vi "drum-seq-pulse-test.vi"() -> ()   [LabVIEW 2019]
uses:
  <vilib>/Rock Robotics/WPI/ThirdParty/JAS_Junk/TrajLib/Enum/DrumSequence_Step_Enum.ctl
  <vilib>/Rock Robotics/WPI/ThirdParty/JAS_Junk/TrajLib/Enum/DrumSequence_State_Enum.ctl
  <vilib>/Rock Robotics/WPI/ThirdParty/JAS_Junk/TrajLib/VI/BoolCmd_Recv_Internal.vi
  <vilib>/Rock Robotics/WPI/ThirdParty/JAS_Junk/TrajLib/VI/DigSeqLogic_Edge_On.vi
  <vilib>/Rock Robotics/WPI/ThirdParty/JAS_Junk/TrajLib/VI/BoolCmd_Send_Internal.vi
  <vilib>/Rock Robotics/WPI/ThirdParty/JAS_Junk/TrajLib/VI/BoolCmd_ObtainQueue.vi
  <vilib>/Rock Robotics/WPI/ThirdParty/JAS_Junk/TrajLib/Trajectory_Library.lvlib
panel:
  out "DrumSeq_State_ENUM":T1
  out "Loop Count":i32
  out "Output 2":bool
  out "Output 1":bool
  out "Error":bool
  out "Ready":bool
  out "Seq  Active":bool
  out "Step Number":T2=enum."Initialize"
  out "can recv":bool
  out "error out 7":errorcluster
  out "error out 6":errorcluster
  in  "seq can cmd":bool
  out "fwd recv":bool
  out "error out 4":errorcluster
  out "error out 2":errorcluster
  in  "milliseconds to wait 2":u32=20
  in  "milliseconds to wait":u32=20
  in  "seq fwd cmd":bool
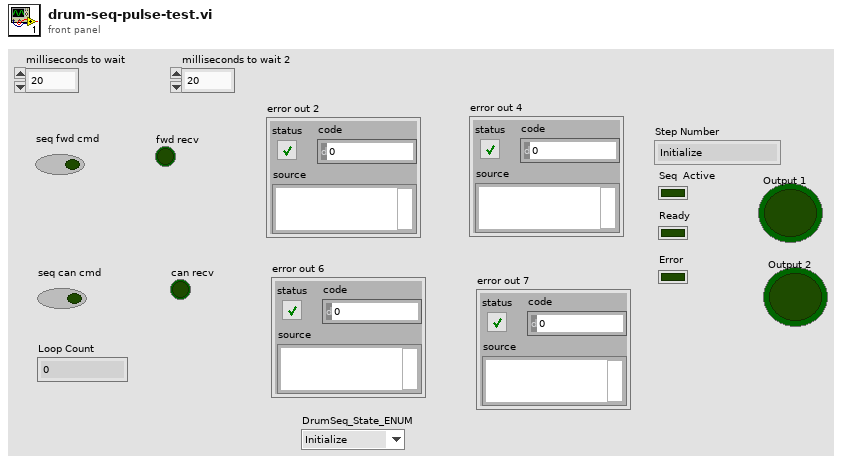
[diagram p1: front panel]
types:
  T1 = typedef "Trajectory_Library.lvlib/DrumSequence_State_Enum.ctl" = enum16{"Initialize", "Ready", "First Step", "Step Wait", "Next State", "Cancel", "Cancel Wait", "Error", "Error Loop"}
  T2 = typedef "Trajectory_Library.lvlib/DrumSequence_Step_Enum.ctl" = enum16{"Do Nothing", "Step 1", "Step 2", "Step 3", "Step 4", "Step 5", "Step 6", "Step 7", "Step 8", "Step 9", "Step 10", "Step 11", "Step 12", "Step 13", "Step 14", "Step 15", "Step 16", "Step 17", "Step 18", "Step 19", "Step 20", "Step 21", "Step 22", "Step 23", "Step 24", "Step 25", "Step 26", "Step 27", "Step 28", "Step 29", "Step 30", "Step 31", "Step 32", "Cancel", "Initialize", "Error"}
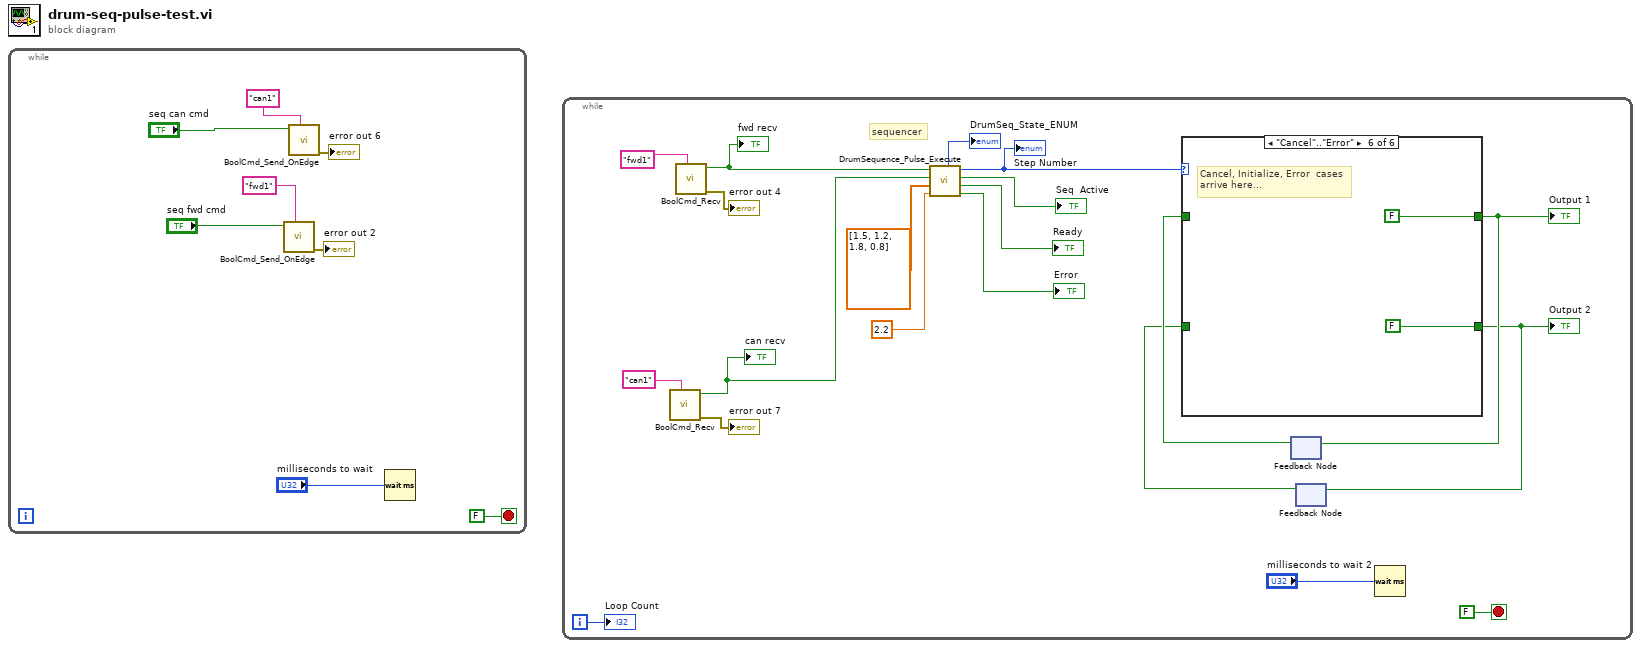
[diagram p0: block diagram]
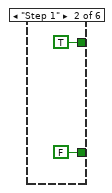
[diagram p3: hidden frame]
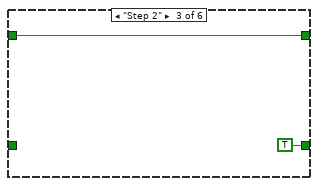
[diagram p4: hidden frame]
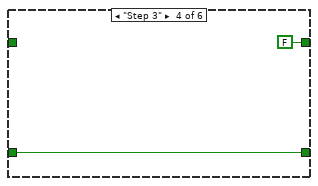
[diagram p5: hidden frame]
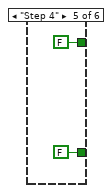
[diagram p6: hidden frame]
diagram:
  n1 = while {
    stop <- FALSE stop-if-true
    n2 = call <vilib>:"BoolCmd_Send_OnEdge.vi"("Command Name"="fwd1", "Value"="seq fwd cmd") -> ("error out"=→"error out 2":errorcluster)  [unwired: 9 in]
    n3 = call <vilib>:"BoolCmd_Send_OnEdge.vi"("Command Name"="can1", "Value"="seq can cmd") -> ("error out"=→"error out 6":errorcluster)  [unwired: 9 in]
    n4 = Wait (ms)(milliseconds to wait="milliseconds to wait") -> ()  [unwired: 1 out]
  }
  n5 = while {
    i -> [w10]
    stop <- FALSE stop-if-true
    # "sequencer"
    n6 = call <vilib>:"BoolCmd_Recv.vi"("Command Name"="can1") -> ("error out"=→"error out 7":errorcluster, "New Request"=w11:bool)  [unwired: 9 in]
    "can recv" <- w11
    n7 = call <vilib>:"BoolCmd_Recv.vi"("Command Name"="fwd1") -> ("error out"=→"error out 4":errorcluster, "New Request"=w24:bool)  [unwired: 9 in]
    "fwd recv" <- w24
    n8 = call <vilib>:"DrumSequence_Pulse_Execute.vi"("Cancel Time Sec"=2.2, "Step Times Sec"=dbl[] [1.5, 1.2, 1.8, 0.8], "Cancel"=w11, "Initiate"=w24) -> ("Error"=→"Error":bool, "Ready"=→"Ready":bool, "Seq  Active"=→"Seq  Active":bool, "Step Number State"=w19:T2, "DrumSeq_State_ENUM"=→"DrumSeq_State_ENUM":T1)  [unwired: 3 in]
    "Step Number" <- w19
    n9 = feedback #1() -> (w13:bool)  [unwired: 1 in]
    n10 = feedback #2() -> (w12:bool)  [unwired: 1 in]
    n11 = case shown="\"Cancel\"..\"Error\"" w19 {
      tunnel: [w30 TRUE w33 FALSE FALSE FALSE] -> w15
      tunnel: [w29 FALSE TRUE w35 FALSE FALSE] -> w14
      tunnel: w13 -> [w30 _ w33 _ _ _]
      tunnel: w12 -> [w29 _ _ w35 _ _]
      frame "Do Nothing", Default {
      }
      frame "Step 1" {
      }
      frame "Step 2" {
      }
      frame "Step 3" {
      }
      frame "Step 4" {
      }
      frame "Cancel".."Error" {
        # "Cancel, Initialize, Error  cases\narrive here..."
      }
    }
    "Output 1" <- w15
    "Output 2" <- w14
    n12 = feedback-in #1(w15) -> ()
    n13 = feedback-in #2(w14) -> ()
    n14 = Wait (ms)(milliseconds to wait="milliseconds to wait 2") -> ()  [unwired: 1 out]
    "Loop Count" <- w10
  }
